vi "fireActionPerformed.vi"(8 "error in (no error)":errorcluster, 10 "Action":T1=enum."BGK Color", 11 "QControl_Graph in":refnum<class "QControl_Graph.lvclass">) -> (0 "error out":errorcluster, 3 "QControl_Graph out":refnum<class "QControl_Graph.lvclass">)   [LabVIEW 2017, in "QControl_Graph.lvclass"]
uses:
  QControl_Graph.lvclass
  Actions.ctl
  QControl_Graph.lvclass/QControl_Graph.ctl
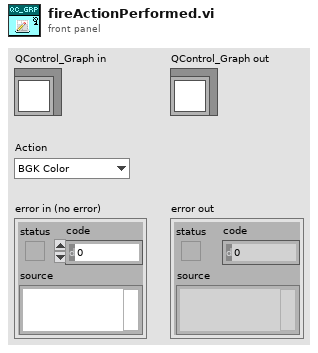
[diagram p1: front panel]
types:
  T1 = typedef "QControl_Graph.lvclass/Actions.ctl" = enum16{"Undefined", "BGK Color", "Highlight Plot", "Mouse Zoom", "Show Cursors", "Cursor Properties", "Show Markers"}
  T2 = typedef "QControl_Graph.lvclass/State Data.ctl" = cluster{"Action Performed":refnum<user-event>, "Show Cursors":bool, "Cursor Properties":T3, "Redraw Cursors":refnum<user-event>}
  T3 = typedef "QControl_Graph.lvclass/Cursor Properties.ctl" = cluster{"Horizontal Line?":bool, "Vertical Line?":bool, "Timestamp":enum16{"at TOP", "at BOTTOM", "none"}, "time format (%H:%M:%S)":string, "size":i16, "font":T4, "alignment(left, top)":T5, "TextFormat":string}
  T4 = typedef "QControl_Graph.lvclass/Font.ctl" = cluster{"Font Name":string, "Size":i16, "Strikeout?":bool, "Italic?":bool, "Underline?":bool, "Outline?":bool, "Shadow":bool, "Bold?":bool}
  T5 = typedef "QControl_Graph.lvclass/Alignment.ctl" = cluster{"Horizontal":T6, "Vertical":T7}
  T6 = typedef "QControl_Graph.lvclass/Alignment.Horizontal.ctl" = enum16{"left", "center", "right"}
  T7 = typedef "QControl_Graph.lvclass/Alignment.Vertical.ctl" = enum16{"top", "center", "bottom"}
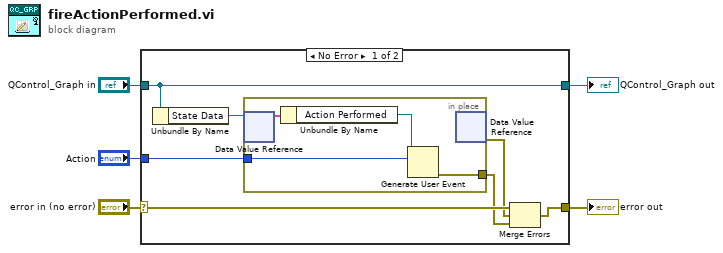
[diagram p0: block diagram]
diagram:
  n1 = case shown="No Error" "error in (no error)" {
    selector: "error in (no error)" -> [w12 w18]
    tunnel: [w8 w18] -> w4
    tunnel: [w11 w17] -> w2
    tunnel: "QControl_Graph in" -> [w11 w17]
    tunnel: "Action" -> [w9 _]
    frame No Error {
      n2 = Unbundle By Name(w11) -> ("State Data"=w10:refnum<data-value>)
      n3 = in-place {
        in-place-border: w9 -> [w14]
        in-place-border: [w13] -> w7
        n4 = in-place-dvr #1(w10) -> (w16:T2)  [unwired: 1 out]
        n5 = Unbundle By Name(w16) -> ("Action Performed"=w15:refnum<user-event>)
        n6 = Generate User Event(user event=w15, event data cluster=w14) -> (error out=w13:errorcluster)  [unwired: 2 in, 1 out]
        n7 = in-place-dvr #1() -> (w6:errorcluster)  [unwired: 1 in, 1 out]
      }
      n8 = Merge Errors(w12, w6, w7) -> (w8:errorcluster)
    }
    frame Error {
    }
  }
  "error out" <- w4
  "QControl_Graph out" <- w2
